vi "Galvo Module.vi"(5 "sample mode":i32(ring)=10178 items=["Finite Samples"=10178, "Continuous Samples"=10123, "Hardware Timed Single Point"=12522], 7 "Action":T1(ring)=enum."Init: Calc scan pattern", 8 "error in (no error)":errorcluster, 10 "System Parameters":T2={"Optical Parameters"={"Obj. Focal Length [mm]"=45.0, "Scan Lens EFL[mm]"=60.0, "Tube Lens EFL[mm]"=180.0, "Galvo V Range (+/-)"=10.0, "Galvo Max Half Angle [Deg]"=19.0, "Max Galvo Range[%]"=0.0}, "Vibratome"={"Z Bottom [mm]"=0.0, "Pre Cut Dwell [s]"=0.0, "Blade Frequency [RPM]"=0, "Slice Speed [mm/s]"=0.0, "Post Cut Dwell [s]"=0.0, "Ramp Time [s]"=0.0, "Start X [mm]"=0.0, "Start Y [mm]"=0.0, "Slice Length [mm]"=0.0, "Slice Axis"=enum."Y Axis", "Controller VISA Ref"="COM4"}, "Table Stages"={"X Stage"={"Position"=0.0, "Is.Enabled?"=FALSE, "Is.Connected?"=FALSE, "Device SN"="45876539", "AccelerationMaximum"=0.0, "VelocityMaximum"=0.0, "Acceleration"=0.0, "Velocity"=0.0, "waitTimeout (ms)"=0, "Model"=enum."None", "Is.Homed?"=FALSE}, "Y Stage"={"Position"=0.0, "Is.Enabled?"=FALSE, "Is.Connected?"=FALSE, "Device SN"="45876539", "AccelerationMaximum"=0.0, "VelocityMaximum"=0.0, "Acceleration"=0.0, "Velocity"=0.0, "waitTimeout (ms)"=0, "Model"=enum."None", "Is.Homed?"=FALSE}, "Z Stage"={"Position"=0.0, "Is.Enabled?"=FALSE, "Is.Connected?"=FALSE, "Device SN"="45876539", "AccelerationMaximum"=0.0, "VelocityMaximum"=0.0, "Acceleration"=0.0, "Velocity"=0.0, "waitTimeout (ms)"=0, "Model"=enum."None", "Is.Homed?"=FALSE}}, "Imaging Parameter"={"Raster Scan Direction"=enum."Uni Directional", "Pixel Dwell Time [Clock Cycles]"=1, "Flyback Time [Clock Cycles]"=10, "XY Center [um]"={"X"=1.0, "Y"=1.0}, "Pixel Step Size [um]"=50.0, "XY Image Size"=enum."256 x 256", "Custom"=TRUE, "Custom Size"={"X"=10, "Y"=10}, "Line Averages"=1}} {"Imaging Parameter"."Line Averages" min=1 max=30 step=1; "Imaging Parameter"."Flyback Time [Clock Cycles]" max=10 step=1; "Imaging Parameter"."Pixel Step Size [um]" min=0.0 max=10.0 step=0.01; "Imaging Parameter"."Custom Size"."Y" min=1 max=30 step=1; "Imaging Parameter"."Custom Size"."X" min=1 max=30 step=1; "Imaging Parameter"."XY Center [um]"."Y" min=1.0 max=30.0 step=1.0; "Imaging Parameter"."XY Center [um]"."X" min=1.0 max=30.0 step=1.0; "Imaging Parameter"."Pixel Dwell Time [Clock Cycles]" max=10 step=1}, 11 "Galvo HW Parameters":T10={"Analog Out Channel"="Dev1/ao0", "Min Voltage"=-5.0, "Max Voltage"=5.0, "Pixel Clock Source"="OnboardClock", "Sample Rate"=1000.0, "Line Clock Out Ch"=""}) -> (0 "error out":errorcluster, 1 "task done?":bool)   [LabVIEW 2018]
uses:
  Controls/System Parameters.ctl
  Controls/Optical Parameters.ctl
  Controls/Vibratome Parameters.ctl
  Controls/Translation Stage Parameters.ctl
  Hardware Mfg/Thorlabs Translation Stages/Controls/Translation Stage Cluster.ctl
  Controls/Translation Stage Types.ctl
  Controls/Imaging Parameters.ctl
  Controls/Scan Direction.ctl
  <vilib>/DAQmx/write.llb/DAQmx Write (Digital 1D U32 1Chan NSamp).vi
  <vilib>/DAQmx/write.llb/DAQmx Write (Analog 2D DBL NChan NSamp).vi
  <vilib>/DAQmx/create/channels.llb/DAQmx Create Channel (DO-Digital Output).vi
  <vilib>/DAQmx/configure/timing.llb/DAQmx Timing (Sample Clock).vi
  <vilib>/DAQmx/create/channels.llb/DAQmx Create Channel (AO-Voltage-Basic).vi
  <vilib>/DAQmx/miscellaneous.llb/DAQmx Fill In Error Info.vi
  <resource>/objmgr/daqmx.rc
panel:
  # "X"
  # "X"
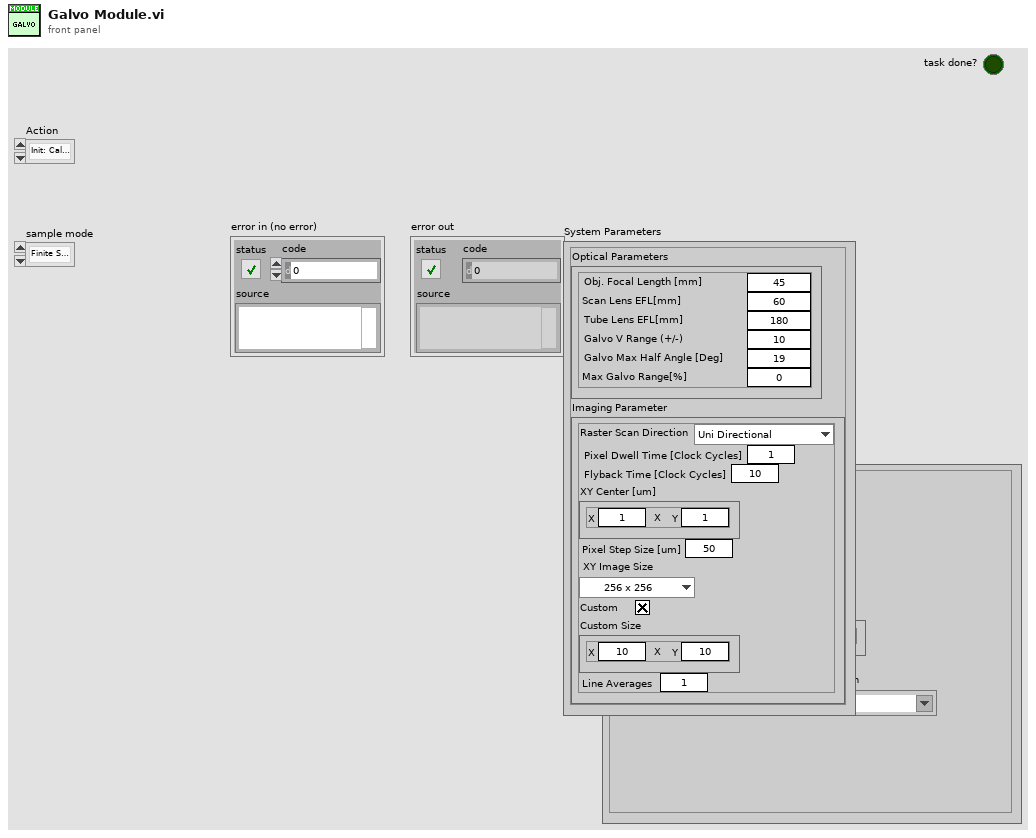
[diagram p1: front panel]
types:
  T1 = enum16{"Configure channels", "Write Scan Pattern", "Start Galvo Task", "Is Task Done?", "Stop Galvo", "Uninit", "Init: Calc scan pattern"}
  T2 = typedef "System Parameters.ctl" = cluster{"Optical Parameters":T3, "Vibratome":T4, "Table Stages":T5, "Imaging Parameter":T8}
  T3 = typedef "Optical Parameters.ctl" = cluster{"Obj. Focal Length [mm]":dbl, "Scan Lens EFL[mm]":dbl, "Tube Lens EFL[mm]":dbl, "Galvo V Range (+/-)":dbl, "Galvo Max Half Angle [Deg]":dbl, "Max Galvo Range[%]":dbl}
  T4 = typedef "Vibratome Parameters.ctl" = cluster{"Z Bottom [mm]":dbl, "Pre Cut Dwell [s]":dbl, "Blade Frequency [RPM]":u16, "Slice Speed [mm/s]":dbl, "Post Cut Dwell [s]":dbl, "Ramp Time [s]":dbl, "Start X [mm]":dbl, "Start Y [mm]":dbl, "Slice Length [mm]":dbl, "Slice Axis":enum16{"X Axis", "Y Axis", "Z Axis"}, "Controller VISA Ref":refnum<visa-resource-name>}
  T5 = typedef "Translation Stage Parameters.ctl" = cluster{"X Stage":T6, "Y Stage":T6, "Z Stage":T6}
  T6 = typedef "Translation Stage Cluster.ctl" = cluster{"Position":dbl, "Is.Enabled?":bool, "Is.Connected?":bool, "Device SN":string, "AccelerationMaximum":dbl, "VelocityMaximum":dbl, "Acceleration":dbl, "Velocity":dbl, "waitTimeout (ms)":i32, "Model":T7, "Is.Homed?":bool}
  T7 = typedef "Translation Stage Types.ctl" = enum16{"None", "Thorlabs LTS", "Thorlabs MLJ"}
  T8 = typedef "Imaging Parameters.ctl" = cluster{"Raster Scan Direction":T9, "Pixel Dwell Time [Clock Cycles]":u16, "Flyback Time [Clock Cycles]":u16, "XY Center [um]":cluster{"X":dbl, "Y":dbl}, "Pixel Step Size [um]":dbl, "XY Image Size":enum16{"32 x 32", "64 x 64", "128 x 128", "256 x 256", "512 x 512", "1024 x 1024", "2048 x 2048"}, "Custom":bool, "Custom Size":cluster{"X":u16, "Y":u16}, "Line Averages":u8}
  T9 = typedef "Scan Direction.ctl" = enum16{"Uni Directional", "Bi Directional", "None"}
  T10 = cluster{"Analog Out Channel":tag, "Min Voltage":dbl, "Max Voltage":dbl, "Pixel Clock Source":tag, "Sample Rate":dbl, "Line Clock Out Ch":tag}
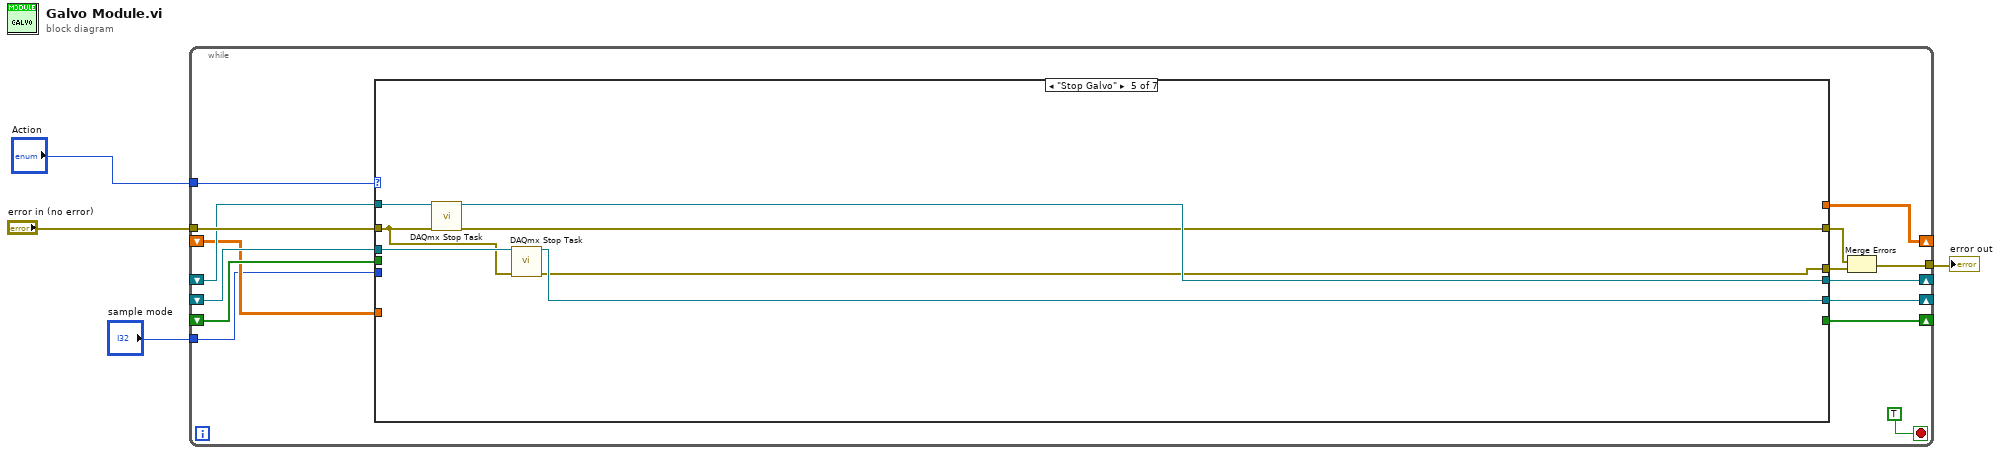
[diagram p0: block diagram]
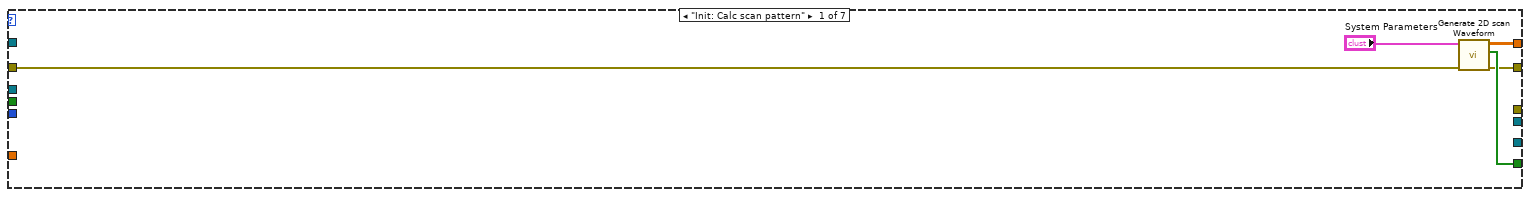
[diagram p2: hidden frame]
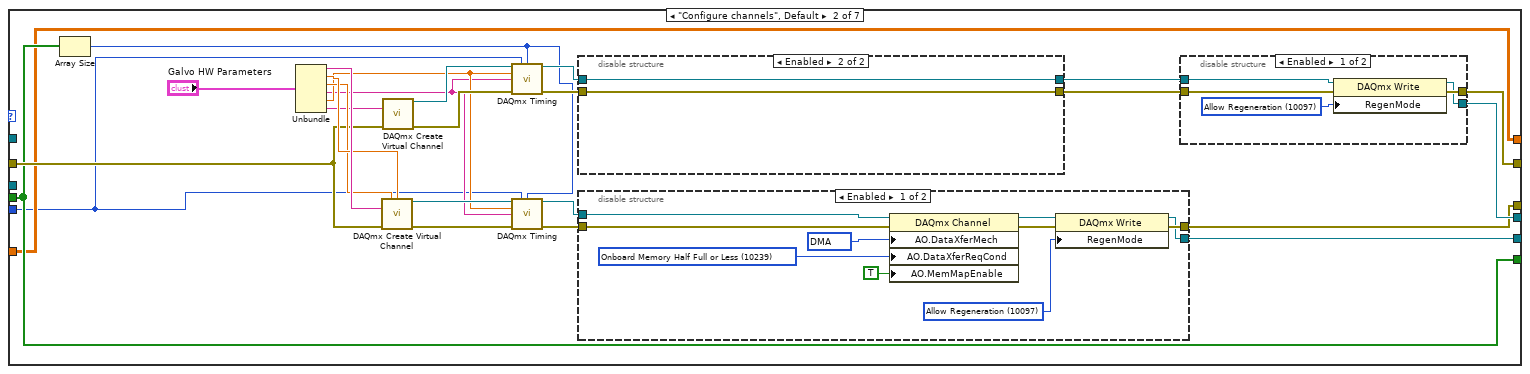
[diagram p3: hidden frame]
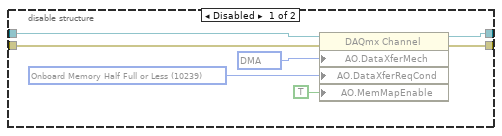
[diagram p6: hidden frame]
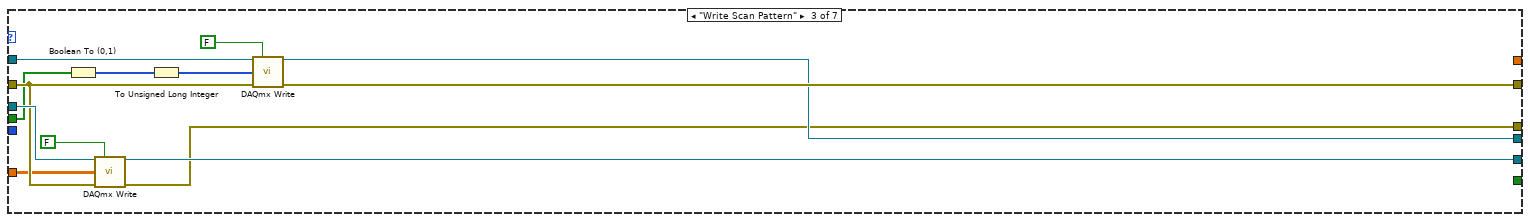
[diagram p7: hidden frame]
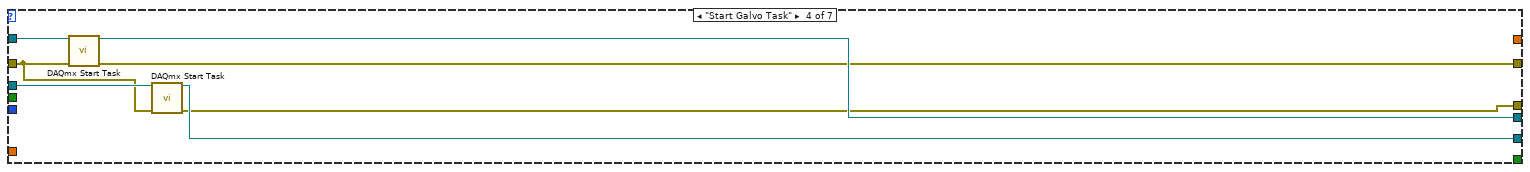
[diagram p8: hidden frame]
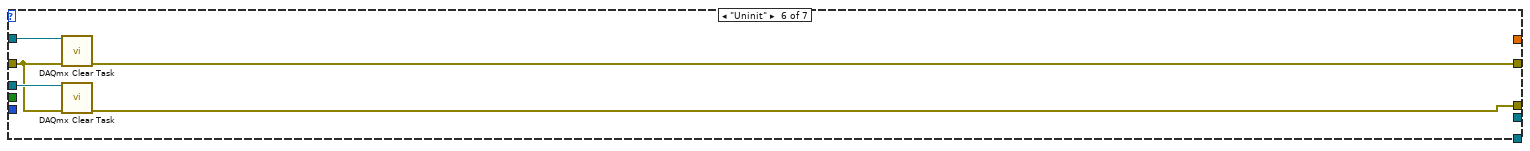
[diagram p9: hidden frame]
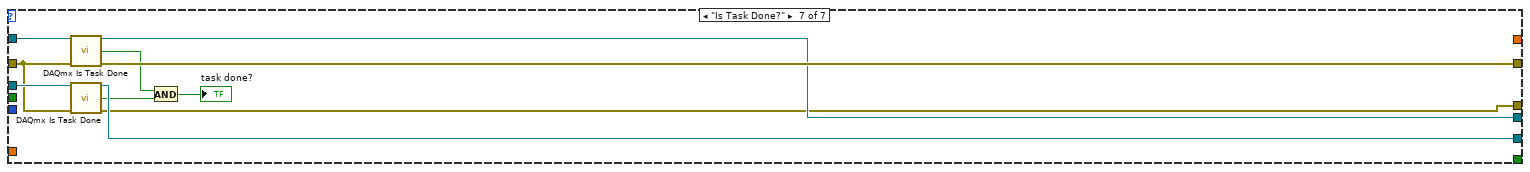
[diagram p10: hidden frame]
diagram:
  n1 = while {
    tunnel: "Action" -> [w19]
    shift-right: [w18] -> _
    shift-left: _ -> [w17]
    tunnel: [w14] -> w3
    tunnel: "error in (no error)" -> [w16]
    shift-right: [w12] -> _
    shift-left: _ -> [w11]
    shift-right: [w10] -> _
    shift-left: _ -> [w7]
    shift-right: [w9] -> _
    shift-left: _ -> [w8]
    tunnel: "sample mode" -> [w6]
    stop <- TRUE stop-if-true
    n2 = case shown="\"Stop Galvo\"" w19 {
      tunnel: [_ w44 w83 w97 w104 _ w119] -> w18
      tunnel: w17 -> [_ _ w91 w98 w105 w110 w120]
      tunnel: w16 -> [w20 w40 w88 w96 w103 w107 w116]
      tunnel: [w22 w32 w87 w93 w100 w109 w115] -> w13
      tunnel: [_ w31 w85 w94 w101 _ w112] -> w12
      tunnel: w11 -> [_ _ w84 w95 w102 w108 w117]
      tunnel: [w24 w28 _ _ _ _ _] -> w10
      tunnel: [w23 w29 _ _ _ _ _] -> w9
      tunnel: w8 -> [_ w29 w82 _ _ _ _]
      tunnel: w7 -> [_ w28 w80 _ _ _ _]
      tunnel: w6 -> [_ w26 _ _ _ _ _]
      tunnel: [_ w25 w79 w92 w99 w106 w111] -> w5
      frame "Init: Calc scan pattern" {
        n3 = call "Generate 2D scan Waveform.vi"("error in (no error)"=w20, "System Parameters [In]"="System Parameters") -> ("error out"=w22:errorcluster, "Digital Line Acq"=w23:bool[], "XY"=w24:dbl[][])  [unwired: 4 in, 3 out]
      }
      frame "Configure channels", Default {
        n4 = Array Size(array=w29) -> (size(s)=w27:i32)
        n5 = Unbundle("Galvo HW Parameters") -> ("Analog Out Channel"=w48:tag, "Min Voltage"=w47:dbl, "Max Voltage"=w46:dbl, "Pixel Clock Source"=w30:tag, "Sample Rate"=w37:dbl, "Line Clock Out Ch"=w43:tag)
        n6 = call-poly <vilib>:"DAQmx Create Virtual Channel.vi"("maximum value"=w46, "minimum value"=w47, "physical channels"=w48, "error in"=w40) -> ("task out"=w42:refnum<k21>, "error out"=w41:errorcluster)  [unwired: 10 in]
        n7 = call-poly <vilib>:"DAQmx Create Virtual Channel.vi"("lines"=w43, "error in"=w40) -> ("task out"=w38:refnum<k21>, "error out"=w39:errorcluster)  [unwired: 12 in]
        n8 = call-poly <vilib>:"DAQmx Timing.vi"("task/channels in"=w38, "sample mode"=w26, "samples per channel"=w27, "rate"=w37, "source"=w30, "error in"=w39) -> ("task out"=w33:refnum<k21>, "error out"=w34:errorcluster)  [unwired: 8 in]
        n9 = call-poly <vilib>:"DAQmx Timing.vi"("task/channels in"=w42, "sample mode"=w26, "samples per channel"=w27, "rate"=w37, "source"=w30, "error in"=w41) -> ("task out"=w45:refnum<k21>, "error out"=w50:errorcluster)  [unwired: 8 in]
        n10 = disable-structure shown="Enabled" {
          disable-tunnel: [w76 w77] -> w36
          disable-tunnel: [w75 w78] -> w35
          disable-tunnel: w34 -> [w71 w78]
          disable-tunnel: w33 -> [w70 w77]
          frame Disabled {
            w73 = 10239 items=["Onboard Memory Empty"=10235, "Onboard Memory Half Full or Less"=10239, "Onboard Memory Less than Full"=10242] ("AO.DataXferReqCond")
            w74 = 10054 items=["DMA"=10054, "Interrupts"=10204, "Programmed I/O"=10264, "USB Bulk"=12590] ("AO.DataXferMech")
            n11 = property class="DAQmx Channel"(reference=w70, error in=w71, "AO.DataXferMech"=w74, "AO.DataXferReqCond"=w73, "AO.MemMapEnable"=TRUE) -> (reference out=w76:refnum<k21>, error out=w75:errorcluster)
          }
          frame Enabled {
          }
        }
        n12 = disable-structure shown="Enabled" {
          disable-tunnel: w50 -> [w67 w68]
          disable-tunnel: w45 -> [w65 w69]
          disable-tunnel: [w61 w68] -> w25
          disable-tunnel: [w58 w69] -> w44
          frame Enabled {
            w59 = 10097 items=["Allow Regeneration"=10097, "Do Not Allow Regeneration"=10158] ("RegenMode")
            w63 = 10239 items=["Onboard Memory Empty"=10235, "Onboard Memory Half Full or Less"=10239, "Onboard Memory Less than Full"=10242] ("AO.DataXferReqCond")
            w64 = 10054 items=["DMA"=10054, "Interrupts"=10204, "Programmed I/O"=10264, "USB Bulk"=12590] ("AO.DataXferMech")
            n13 = property class="DAQmx Channel"(reference=w65, error in=w67, "AO.DataXferMech"=w64, "AO.DataXferReqCond"=w63, "AO.MemMapEnable"=TRUE) -> (reference out=w60:refnum<k21>, error out=w66:errorcluster)
            n14 = property class="DAQmx Write"(reference=w60, error in=w66, "RegenMode"=w59) -> (reference out=w58:refnum<k21>, error out=w61:errorcluster)
          }
          frame Disabled {
          }
        }
        n15 = disable-structure shown="Enabled" {
          disable-tunnel: w36 -> [w55 w57]
          disable-tunnel: w35 -> [w54 w56]
          disable-tunnel: [w52 w56] -> w32
          disable-tunnel: [w51 w57] -> w31
          frame Enabled {
            w53 = 10097 items=["Allow Regeneration"=10097, "Do Not Allow Regeneration"=10158] ("RegenMode")
            n16 = property class="DAQmx Write"(reference=w55, error in=w54, "RegenMode"=w53) -> (reference out=w51:refnum<k21>, error out=w52:errorcluster)
          }
          frame Disabled {
          }
        }
      }
      frame "Write Scan Pattern" {
        n17 = Boolean To (0,1)(Boolean=w82) -> (0, 1=w89:i16[])
        n18 = call-poly <vilib>:"DAQmx Write.vi"("task/channels in"=w91, "auto start"=FALSE, "data"=w80, "error in"=w88) -> ("task out"=w83:refnum<k21>, "error out"=w79:errorcluster)  [unwired: 9 in, 1 out]
        n19 = To Unsigned Long Integer(number=w89) -> (unsigned 32bit integer=w81:u32[])
        n20 = call-poly <vilib>:"DAQmx Write.vi"("task/channels in"=w84, "auto start"=FALSE, "data"=w81, "error in"=w88) -> ("task out"=w85:refnum<k21>, "error out"=w87:errorcluster)  [unwired: 9 in, 1 out]
      }
      frame "Start Galvo Task" {
        n21 = call <vilib>:"DAQmx Start Task.vi"("task/channels in"=w95, "error in"=w96) -> ("task out"=w94:refnum<k21>, "error out"=w93:errorcluster)  [unwired: 12 in]
        n22 = call <vilib>:"DAQmx Start Task.vi"("task/channels in"=w98, "error in"=w96) -> ("task out"=w97:refnum<k21>, "error out"=w92:errorcluster)  [unwired: 12 in]
      }
      frame "Stop Galvo" {
        n23 = call <vilib>:"DAQmx Stop Task.vi"("task/channels in"=w102, "error in"=w103) -> ("task out"=w101:refnum<k21>, "error out"=w100:errorcluster)  [unwired: 12 in]
        n24 = call <vilib>:"DAQmx Stop Task.vi"("task/channels in"=w105, "error in"=w103) -> ("task out"=w104:refnum<k21>, "error out"=w99:errorcluster)  [unwired: 12 in]
      }
      frame "Uninit" {
        n25 = call <vilib>:"DAQmx Clear Task.vi"("task in"=w108, "error in"=w107) -> ("error out"=w109:errorcluster)  [unwired: 13 in]
        n26 = call <vilib>:"DAQmx Clear Task.vi"("task in"=w110, "error in"=w107) -> ("error out"=w106:errorcluster)  [unwired: 13 in]
      }
      frame "Is Task Done?" {
        n27 = call <vilib>:"DAQmx Is Task Done.vi"("task/channels in"=w117, "error in"=w116) -> ("task out"=w112:refnum<k21>, "task done?"=w113:bool, "error out"=w115:errorcluster)  [unwired: 11 in]
        n28 = call <vilib>:"DAQmx Is Task Done.vi"("task/channels in"=w120, "error in"=w116) -> ("task out"=w119:refnum<k21>, "task done?"=w118:bool, "error out"=w111:errorcluster)  [unwired: 11 in]
        n29 = And(x=w113, y=w118) -> (x .and. y?=→"task done?":bool)
      }
    }
    n30 = Merge Errors(w13, w5) -> (w14:errorcluster)
  }
  "error out" <- w3
